vi "Load Configuration.vi"(8 "error in (no error)":errorcluster, 11 "Configuration in":refnum<class "Configuration.lvclass">) -> (0 "error out":errorcluster, 3 "Configuration out":refnum<class "Configuration.lvclass">)   [LabVIEW 2023, in "Configuration.lvlib" / "Configuration.lvclass"]
doc: "Read config.ini file in to the configuration map for reference"
uses:
  Library/Configuration.lvclass
  Library/Configuration.lvclass/Configuration.ctl
  <vilib>/Utility/config.llb/NI_LVConfig.lvlib
  Custom Controls/Config.ctl
  Custom Controls/Definitions.ctl
  <vilib>/Utility/config.llb/Read Key (String).vi
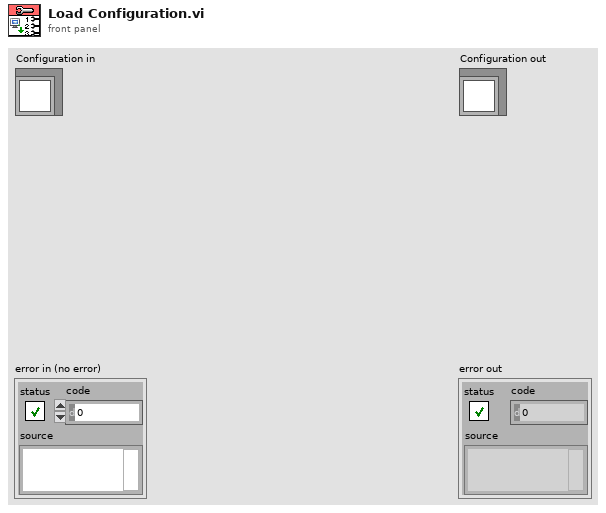
[diagram p1: front panel]
types:
  T1 = typedef "Configuration.lvlib/Configuration.lvclass/Definitions.ctl" = map{string, T2}
  T2 = typedef "Configuration.lvlib/Configuration.lvclass/Config.ctl" = map{string, string}
  T3 = typedef "NI_LVConfig.lvlib/Config Data RefNum.ctl" = refnum<k1>
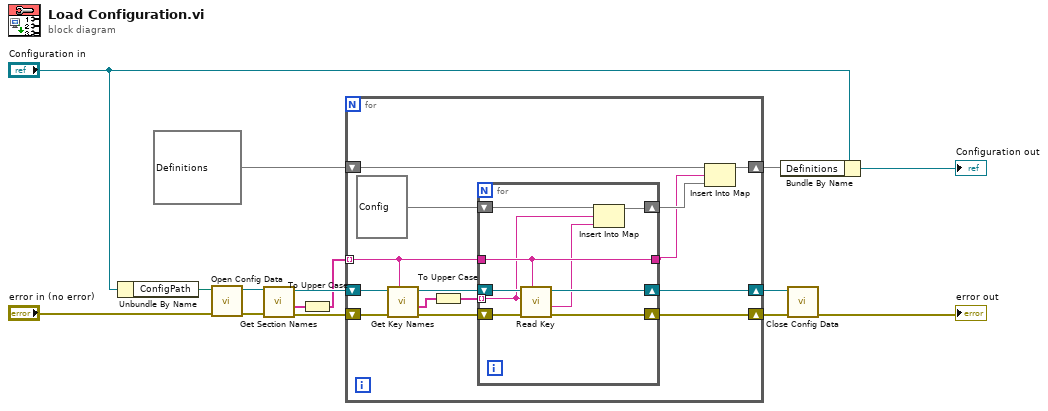
[diagram p0: block diagram]
diagram:
  n1 = Unbundle By Name("Configuration in") -> ("ConfigPath"=w2:path)
  n2 = call <vilib>:"Open Config Data.vi"("error in (no error)"="error in (no error)", "configuration file path"=w2) -> ("error out"=w14:errorcluster, "refnum"=w15:T3)  [unwired: 7 in, 1 out]
  n3 = call <vilib>:"Get Section Names.vi"("error in (no error)"=w14, "refnum"=w15) -> ("error out"=w10:errorcluster, "section names"=w13:string[], "refnum out"=w11:T3)  [unwired: 7 in]
  n4 = To Upper Case(1:w13) -> (0:w1:string[])
  n5 = for {
    tunnel: w1 -> [w25] mode=indexing
    shift-right: [w22] -> w7
    shift-left: w11 -> [w28]
    shift-right: [w23] -> w8
    shift-left: w10 -> [w29]
    shift-right: [w19] -> w4
    shift-left: T1 {} ("Definitions") -> [w20]
    n6 = call <vilib>:"Get Key Names.vi"("section"=w25, "error in (no error)"=w29, "refnum"=w28) -> ("error out"=w26:errorcluster, "key names"=w24:string[], "refnum out"=w27:T3)  [unwired: 5 in, 1 out]
    n7 = To Upper Case(1:w24) -> (0:w16:string[])
    n8 = for {
      shift-right: [w35] -> w22
      shift-left: w27 -> [w36]
      shift-right: [w38] -> w23
      shift-left: w26 -> [w37]
      tunnel: w25 -> [w34]
      tunnel: [w34] -> w17
      tunnel: w16 -> [w31] mode=indexing
      shift-right: [w32] -> w18
      shift-left: T2 {} ("Config") -> [w33]
      n9 = call-poly <vilib>:"Read Key.vi"("section"=w34, "error in (no error)"=w37, "key"=w31, "refnum"=w36) -> ("error out"=w38:errorcluster, "value"=w30:string, "refnum out"=w35:T3)  [unwired: 4 in, 1 out]
      n10 = Insert Into Map(map in=w33, key=w31, value=w30) -> (map out=w32:T2)  [unwired: 2 out]
    }
    n11 = Insert Into Map(map in=w20, key=w17, value=w18) -> (map out=w19:T1)  [unwired: 2 out]
  }
  n12 = Bundle By Name(cluster="Configuration in", "Definitions"=w4) -> (→"Configuration out":refnum<class "Configuration.lvclass">)
  n13 = call <vilib>:"Close Config Data.vi"("error in (no error)"=w8, "refnum"=w7) -> ("error out"=→"error out":errorcluster)  [unwired: 8 in, 1 out]
